vi "ST example Set Speed.vi"() -> ()   [LabVIEW 2009]
panel:
  in  "New Speed":string="1000"
  out "Motor Speed":string
  out "STATUS\nREADY":bool
  out "SET\nSPEED":bool
  out "GOT\nSPEED":bool
  # "THIS IS A TEST ROUTINE FOR THE GETTING AND SETTING OF \nMOTOR SPEEDS"
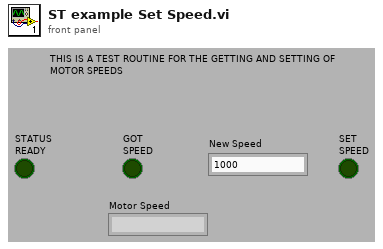
[diagram p1: front panel]
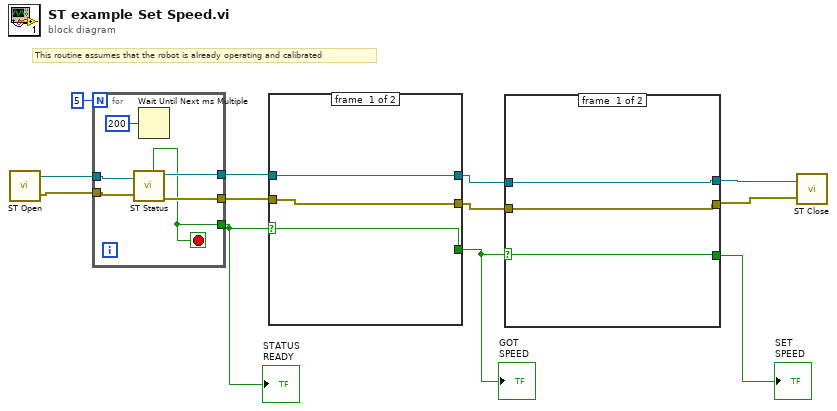
[diagram p0: block diagram]
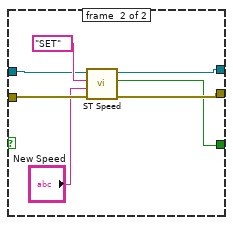
[diagram p2: hidden frame]
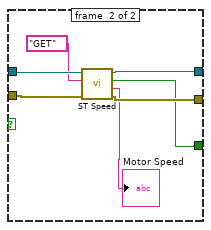
[diagram p3: hidden frame]
diagram:
  # "This routine assumes that the robot is already operating and calibrated"
  n1 = call "ST Open.vi"() -> ("VISA resource name out"=w9:refnum<visa-resource-name>, "error out"=w8:errorcluster)  [unwired: 1 in]
  n2 = for {
    N: 5 -> [_]
    tunnel: w9 -> [w17]
    tunnel: w8 -> [w18]
    tunnel: [w16] -> w6
    tunnel: [w15] -> w5
    tunnel: [w13] -> w7
    stop <- w13 stop-if-true
    n3 = call "ST Status.vi"("error in (no error)"=w18, "VISA resource name"=w17) -> ("error out"=w16:errorcluster, "VISA resource name out"=w15:refnum<visa-resource-name>, "Ready and OK"=w13:bool)  [unwired: 2 out]
    n4 = Wait Until Next ms Multiple(millisecond multiple=u32 200) -> ()  [unwired: 1 out]
  }
  "STATUS\nREADY" <- w7
  n5 = case shown="True" w7 {
    selector: w7 -> [w19 _]
    tunnel: w5 -> [w21 w28]
    tunnel: w6 -> [w20 w27]
    tunnel: [w21 w26] -> w12
    tunnel: [w20 w25] -> w4
    tunnel: [w19 w24] -> w11
    frame #0 {
    }
    frame #1 {
      n6 = call "ST Speed.vi"("error in (error out)"=w27, "Action"="GET", "VISA resource name in"=w28) -> ("error out"=w25:errorcluster, "Motor Speed"=→"Motor Speed":string, "Complete"=w24:bool, "VISA resource name out"=w26:refnum<visa-resource-name>)  [unwired: 1 in]
    }
  }
  "GOT\nSPEED" <- w11
  n7 = case shown="True" w11 {
    selector: w11 -> [w29 _]
    tunnel: w12 -> [w31 w37]
    tunnel: w4 -> [w30 w36]
    tunnel: [w31 w35] -> w2
    tunnel: [w30 w34] -> w1
    tunnel: [w29 w33] -> w3
    frame #0 {
    }
    frame #1 {
      n8 = call "ST Speed.vi"("error in (error out)"=w36, "New Speed"="New Speed", "Action"="SET", "VISA resource name in"=w37) -> ("error out"=w34:errorcluster, "Complete"=w33:bool, "VISA resource name out"=w35:refnum<visa-resource-name>)  [unwired: 1 out]
    }
  }
  "SET\nSPEED" <- w3
  n9 = call "ST Close.vi"("error in (no error)"=w1, "VISA resource name"=w2) -> ()
